vi "TDMS Express Read Data (Time Domain).vi"() -> ()   [LabVIEW 2023]
doc: "This example demonstrates how to read data from a TDMS file using the Read From Measurement File Express VI."
panel:
  out "Element number":i32
  out "Signals":dynamicdata(graph)
  # "Overview: Demonstrates how to read data from a .tdms file using the Read From Measurement File Express VI.\nInstructions:\n1. Make sure you have already run TDMS Express Write Data (Time Domain).vi.\n2. Run the VI. \n3. Delete the .tdms file (located at [LabVIEW Data]\\Example Time Domain.tdms) when you are done."
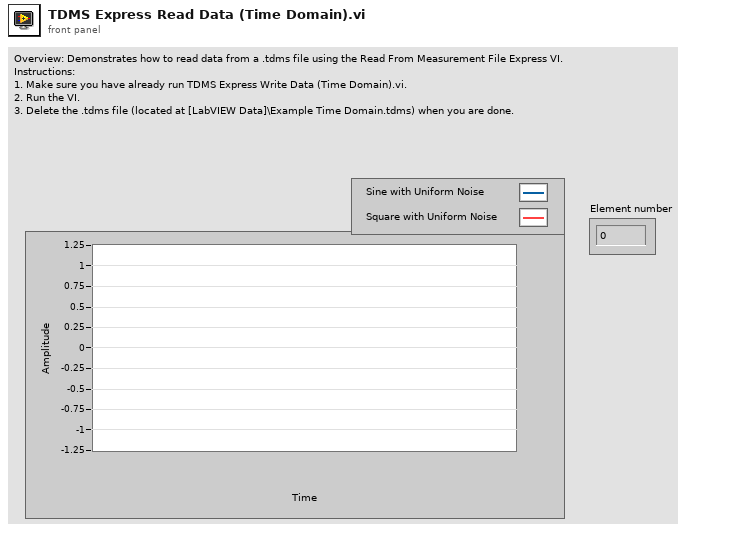
[diagram p1: front panel]
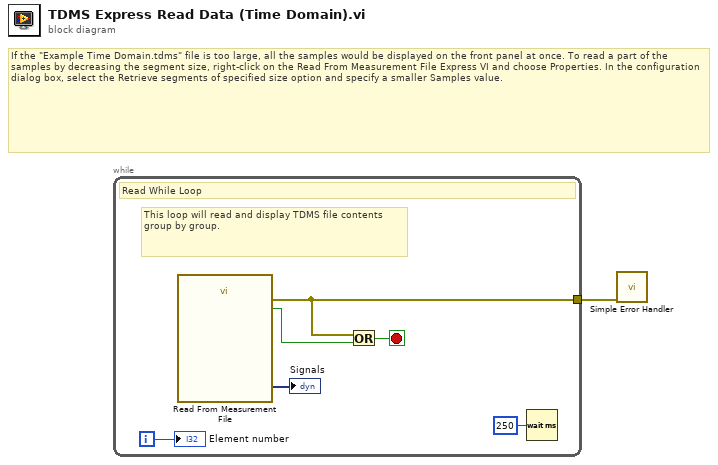
[diagram p0: block diagram]
diagram:
  # "If the \"Example Time Domain.tdms\" file is too large, all the samples would be displayed on the front panel at once. To read a part of the samples by decreasing the segment size, right-click on the Read From Measurement File Express VI and choose Properties. In the configuration dialog box, select the Retrieve segments of specified size option and specify a smaller Samples value."
  n1 = while {
    tunnel: [w2] -> w1
    i -> [w6]
    stop <- w3 stop-if-true
    # "This loop will read and display TDMS file contents group by group."
    # "Read While Loop"
    n2 = call "Read From Measurement File"() -> ("error out"=w2:errorcluster, "Signals"=→"Signals":dynamicdata, "EOF?"=w7:bool)  [unwired: 6 in, 3 out]
    n3 = Or(x=w2, y=w7) -> (x .or. y?=w3:bool)
    n4 = Wait (ms)(milliseconds to wait=u32 250) -> ()  [unwired: 1 out]
    "Element number" <- w6
  }
  n5 = call <vilib>:"Simple Error Handler.vi"("error in (no error)"=w1) -> ()  [unwired: 4 in, 5 out]
